vi "struct_ads_vol_dW_dA_ARho.vi"(8 "Error (Input)":errorcluster, 9 "Saturated liquid density of adsorpt rho_l in kg/m3 (Input)":dbl, 10 "Adsorption potential A in J/mol (Input)":dbl, 11 "Reference working pair (Input)":i64) -> (0 "Error (Output)":errorcluster caption="Error(Output)", 3 "Der. of volumetric loading wrt. adsorption potential in m3mol/kg/J (Output)":dbl)   [LabVIEW 2017]
doc: "ads_vol_dW_dA_ARho:\n * -------------------\n *\n * Calculates derivative of equilibrium volumetric loading dW_dA in młmol/kg/J\n * depending on equilibrium adsorption potential A in J/mol and saturated liquid\n * density of adsorpt rho_l in kg/m3.\n *\n * Parameters:\n * -----------\n * double A_Jmol:\n * Equilibrium adsorption potential A in mol/J.\n * double rho_l_kgm3:\n * Saturated liquid density of adsorpt rho_l in kg/m3.\n * struct *WorkingPair:\n * Pointer of WorkingPair-struct.\n *\n * Returns:\n * --------\n * double:\n * Derivative of volumetric loading wrt. adsorption potential in\n * młmol/kg/J.\n *\n * Remarks:\n * --------\n * This function is only valid for isotherm models based on the volumetric\n * approach.\n * Saturated liquid density of adsorpt is required to calculate volumetric\n * loading from characteristic curve in m3/kg when coefficients would directly\n * return loading w in kg/kg.\n *\n * History:\n * --------\n * 07/13/2021, by Jannik Driesel (supervised by Mirko Engelpracht):\n * First implementation."
uses:
  data/win32bit/libsorpPropLib.dll
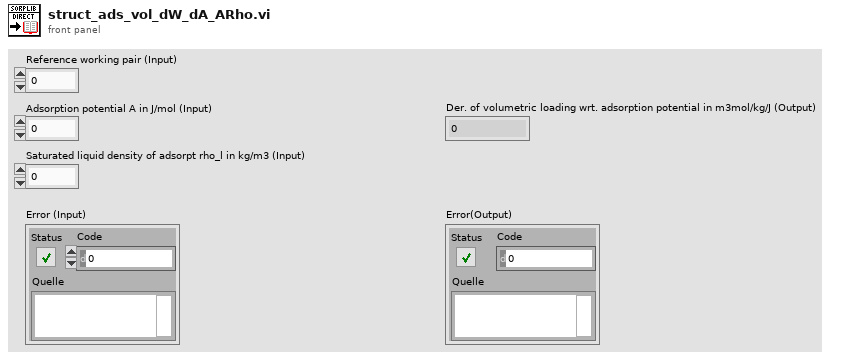
[diagram p1: front panel]
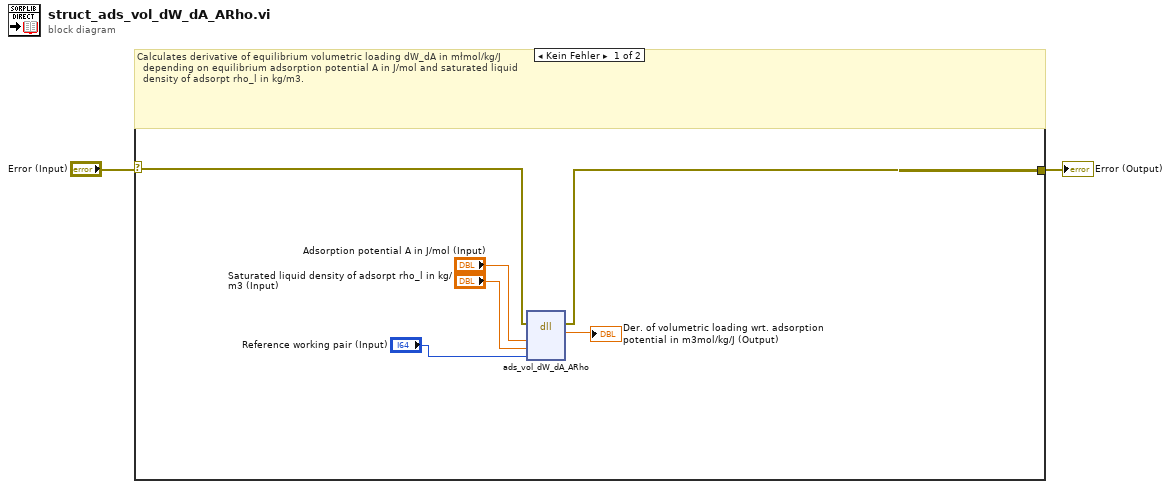
[diagram p0: block diagram]
diagram:
  n1 = case shown="Kein Fehler" "Error (Input)" {
    selector: "Error (Input)" -> [w7 w9]
    tunnel: [w6 w9] -> w1
    frame No Error {
      # "Calculates derivative of equilibrium volumetric loading dW_dA in młmol/kg/J\n  depending on equilibrium adsorption potential A in J/mol and saturated liquid\n  density of adsorpt rho_l in kg/m3."
      n2 = dll-call lib="D:/Driesel/SorpLibLocal/LabVIEW_wrapper/data/win32bit/libsorpPropLib.dll" fn="ads_vol_dW_dA_ARho"(error in=w7, "A_Jmol"="Adsorption potential A in J/mol (Input)", "rho_l_kgm3"="Saturated liquid density of adsorpt rho_l in kg/m3 (Input)", "workingPair"="Reference working pair (Input)") -> (error out=w6:errorcluster, "dW_dA_m3molkgJ"=→"Der. of volumetric loading wrt. adsorption potential in m3mol/kg/J (Output)":dbl)  [unwired: 5 in, 1 out]
    }
    frame Error {
      # "Error - No calculations"
    }
  }
  "Error (Output)" <- w1
